vi "start.vi"(8 "error in (no error)":errorcluster, 11 "niDAQmxAO in":refnum<class "niDAQmxAO.lvclass">) -> (0 "error out":errorcluster, 3 "niDAQmxAO out":refnum<class "niDAQmxAO.lvclass">)   [LabVIEW 2009, in "Hardware.lvlib" / "Channels.lvlib" / "niDAQmxAO.lvclass"]
uses:
  niDAQmxAO.lvclass
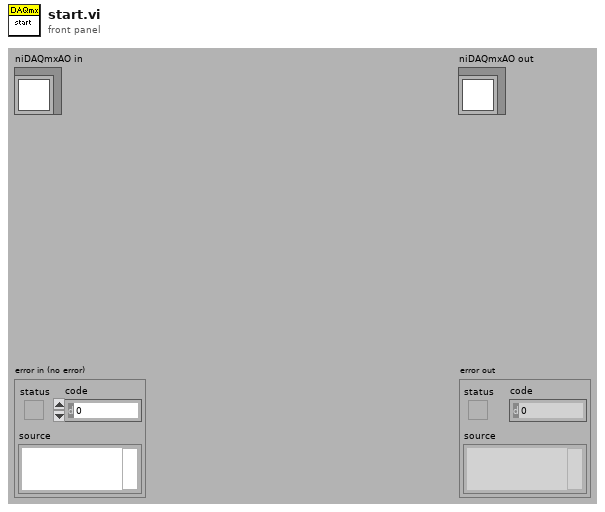
[diagram p1: front panel]
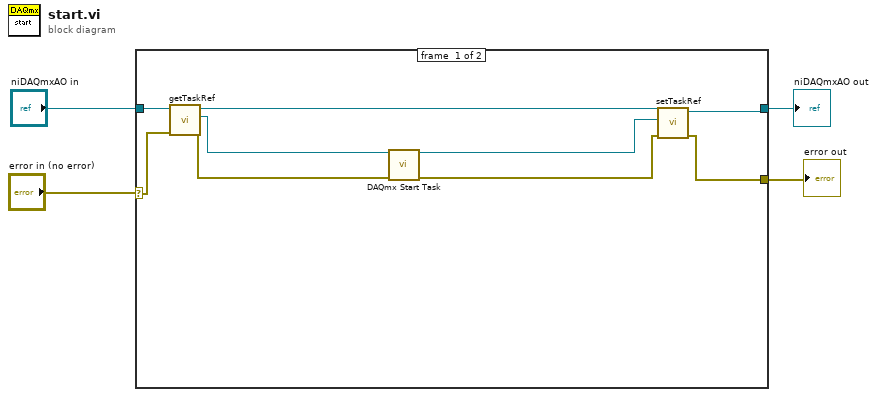
[diagram p0: block diagram]
diagram:
  n1 = case shown="No Error" "error in (no error)" {
    selector: "error in (no error)" -> [w12 w15]
    tunnel: [w9 w15] -> w3
    tunnel: [w10 w14] -> w1
    tunnel: "niDAQmxAO in" -> [w13 w14]
    frame #0 {
      n2 = call "getTaskRef.vi"("error in (no error)"=w12, "niDAQmxAO.lvclass in"=w13) -> ("error out"=w5:errorcluster, "DAQmx Task Ref"=w6:refnum<k21>, "niDAQmxAO.lvclass out"=w7:refnum<class "niDAQmxAO.lvclass">)  [unwired: 7 in]
      n3 = call <vilib>:"DAQmx Start Task.vi"("task/channels in"=w6, "error in"=w5) -> ("task out"=w11:refnum<k21>, "error out"=w8:errorcluster)  [unwired: 12 in]
      n4 = call "setTaskRef.vi"("error in (no error)"=w8, "DAQmx Task Ref"=w11, "niDAQmxAO.lvclass in"=w7) -> ("error out"=w9:errorcluster, "niDAQmxAO.lvclass out"=w10:refnum<class "niDAQmxAO.lvclass">)  [unwired: 7 in]
    }
    frame #1 {
    }
  }
  "error out" <- w3
  "niDAQmxAO out" <- w1
